vi "Autobuild Main.vi"() -> ()   [LabVIEW 2021]
uses:
  subVIs/Package Builder API/build type.ctl
  subVIs/Package Builder API/NI Package Builder API.lvlib
panel:
  out "command line standard output":string
  in  "package builder solution path":path=path "C:/dev/class-d-amplifier/package/ClassDAmplifier.pbs"
  in  "Projects":path[](array[path])=[path "C:/dev/class-d-amplifier/source/crosstalk/Crosstalk_Class D Amplifier.lvproj", path "C:/dev/class-d-amplifier/source/single tone/Single Tone Measurements_Class D Amplifier.lvproj", path "C:/dev/class-d-amplifier/source/stepped frequency sweep/Stepped Frequency Sweep_Class D Amplifier.lvproj", path "C:/dev/class-d-amplifier/source/efficiency/Efficiency_Class D Amplifier.lvproj", path "C:/dev/class-d-amplifier/source/efficiency sweep/Efficiency Sweep_Class D Amplifier.lvproj"]
  in  "error in (no error)":errorcluster
  out "error out":errorcluster
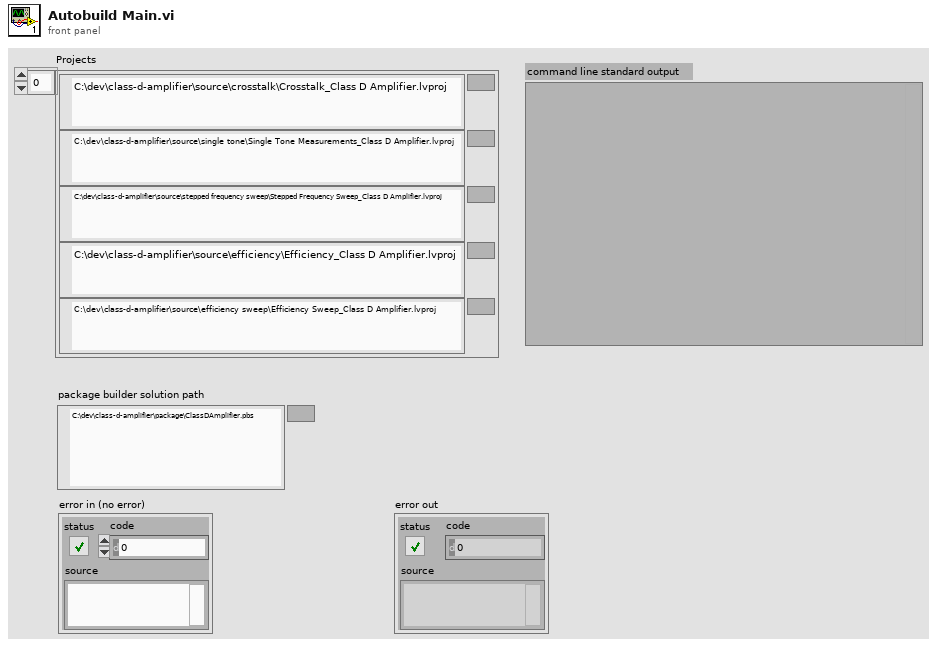
[diagram p1: front panel]
types:
  T1 = typedef "NI Package Builder API.lvlib/build type.ctl" = enum16{"packages", "feeds", "solution"}
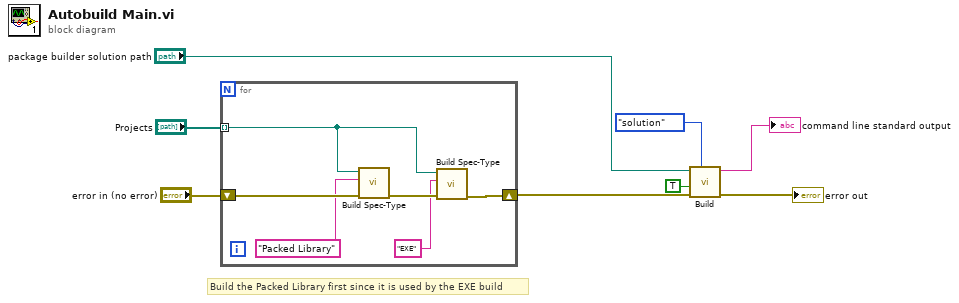
[diagram p0: block diagram]
diagram:
  # "Build the Packed Library first since it is used by the EXE build"
  n1 = for {
    shift-right: [w10] -> w6
    shift-left: "error in (no error)" -> [w14]
    tunnel: "Projects" -> [w9] mode=indexing
    n2 = call "Build Spec-Type.vi"("error in (no error)"=w14, "Type"="Packed Library", "Path to project"=w9) -> ("error out"=w13:errorcluster)  [unwired: 8 in]
    n3 = call "Build Spec-Type.vi"("error in (no error)"=w13, "Type"="EXE", "Path to project"=w9) -> ("error out"=w10:errorcluster)  [unwired: 8 in]
  }
  n4 = call "Build.vi"("bulid type"=build_type."solution", "error in (no error)"=w6, "save build info to solution"=TRUE, "package builder solution path"="package builder solution path") -> ("error out"=→"error out":errorcluster, "command line standard output"=→"command line standard output":string)  [unwired: 6 in]
